vi "GetProduct.vi"(8 "error in (no error)":errorcluster, 11 "PizzaBuilder(Builder) in":refnum<class "PizzaBuilder(Builder).lvclass">) -> (0 "error out":errorcluster, 2 "Pizza":refnum<class "Pizza(Product).lvclass">, 3 "PizzaBuilder(Builder) out":refnum<class "PizzaBuilder(Builder).lvclass">)   [LabVIEW 2014, in "PizzaBuilder(Builder).lvclass"]
uses:
  PizzaBuilder(Builder).lvclass
  Pizza(Product)/Pizza(Product).lvclass
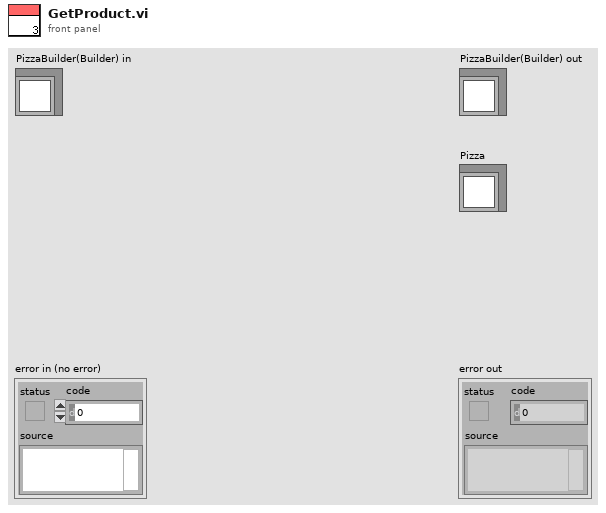
[diagram p1: front panel]
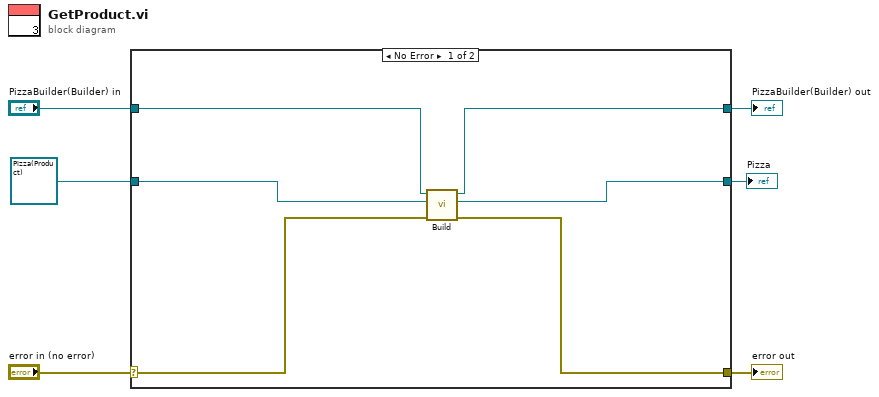
[diagram p0: block diagram]
diagram:
  n1 = case shown="No Error" "error in (no error)" {
    selector: "error in (no error)" -> [w8 w15]
    tunnel: [w7 w15] -> w5
    tunnel: [w10 w14] -> w3
    tunnel: "PizzaBuilder(Builder) in" -> [w11 w14]
    tunnel: refnum<class "Pizza(Product).lvclass"> refnum ("Pizza") -> [w12 w13]
    tunnel: [w9 w13] -> w1
    frame No Error {
      n2 = call-dynamic "Build.vi"("error in (no error)"=w8, "Pizza"=w12, "PizzaBuilder(Builder) in"=w11) -> ("error out"=w7:errorcluster, "Pizza out"=w9:refnum<class "Pizza(Product).lvclass">, "PizzaBuilder(Builder) out"=w10:refnum<class "PizzaBuilder(Builder).lvclass">)  [unwired: 6 in]
    }
    frame Error {
    }
  }
  "error out" <- w5
  "PizzaBuilder(Builder) out" <- w3
  "Pizza" <- w1
